vi "VI Tree.vi"   [LabVIEW 2013]
uses:
  Action/OUTPUT(General).vi
  Action/RESET(General).vi
  Configure/SetPower(General).vi
  Configure/SetVoltRange(General).vi
  Configure/SetCurrent(General).vi
  Configure/SetFrequency(General).vi
  Configure/SetVoltage(General).vi
  Data/ReadVoltageSetting(General).vi
  Data/ReadFrequencySetting(General).vi
  Data/ReadCurrentSetting(General).vi
  Data/ReadPowerSetting(General).vi
panel:
  # "(c) 2017 Preen AC Source Interument.  ALL RIGHTS RESERVED."
  # "SEE DIAGRAM\nFOR VI TREE."
  # "Version 1.00"
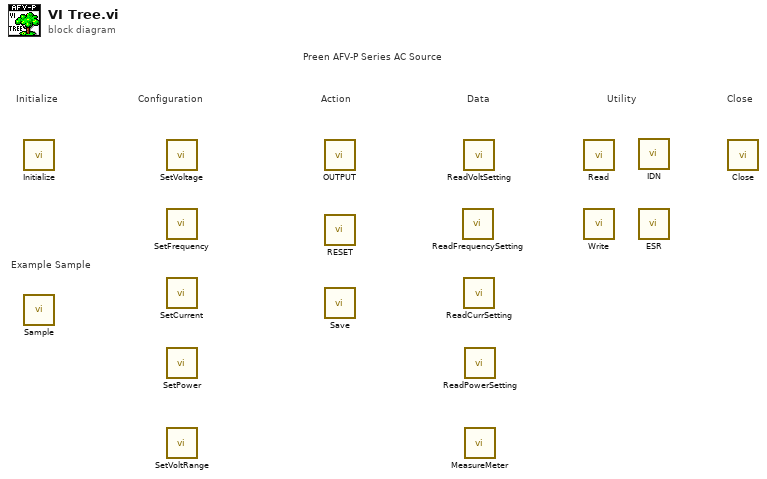
[diagram p0: block diagram]
diagram:
  # "Example Sample"
  # "Preen AFV-P Series AC Source"
  # "Configuration"
  # "Utility"
  # "Data"
  # "Action"
  # "Close"
  # "Initialize"
  n1 = call "Initialize.vi"() -> ()  [unwired: 10 in, 2 out]
  n2 = call "Sample.vi"() -> ()  [unwired: 12 in]
  n3 = call-poly "SetVoltage.vi"() -> ()  [unwired: 10 in, 2 out]
  n4 = call-poly "SetFrequency.vi"() -> ()  [unwired: 10 in, 2 out]
  n5 = call-poly "SetCurrent.vi"() -> ()  [unwired: 10 in, 2 out]
  n6 = call-poly "SetPower.vi"() -> ()  [unwired: 10 in, 2 out]
  n7 = call-poly "SetVoltRange.vi"() -> ()  [unwired: 10 in, 2 out]
  n8 = call-poly "OUTPUT.vi"() -> ()  [unwired: 10 in, 2 out]
  n9 = call-poly "RESET.vi"() -> ()  [unwired: 10 in, 2 out]
  n10 = call "Save.vi"() -> ()  [unwired: 10 in, 2 out]
  n11 = call-poly "ReadFrequencySetting.vi"() -> ()  [unwired: 9 in, 3 out]
  n12 = call-poly "ReadVoltSetting.vi"() -> ()  [unwired: 9 in, 3 out]
  n13 = call-poly "ReadCurrSetting.vi"() -> ()  [unwired: 9 in, 3 out]
  n14 = call-poly "ReadPowerSetting.vi"() -> ()  [unwired: 9 in, 3 out]
  n15 = call "MeasureMeter.vi"() -> ()  [unwired: 9 in, 3 out]
  n16 = call "Read.vi"() -> ()  [unwired: 9 in, 3 out]
  n17 = call "Write.vi"() -> ()  [unwired: 10 in, 2 out]
  n18 = call "IDN.vi"() -> ()  [unwired: 9 in, 3 out]
  n19 = call "ESR.vi"() -> ()  [unwired: 10 in, 2 out]
  n20 = call "Close.vi"() -> ()  [unwired: 11 in, 1 out]
